vi "HW_Gantner_Parse Construct Default Modu Configuration.vi"(5 "Chan dflt Para in":T5, 7 "DevInfo":T1, 11 "ModuCFG from File":T2) -> (3 "ModuCFG out":T2)   [LabVIEW 2016]
uses:
  Ctrls/HardWare _ Module Configuration.ctl
  Ctrls/HardWare _ Channel Configurations PopUp Type.ctl
  ToolKit/Popup/Private/Ctrls/POP_Data Type.ctl
  Gantner Device Info.ctl
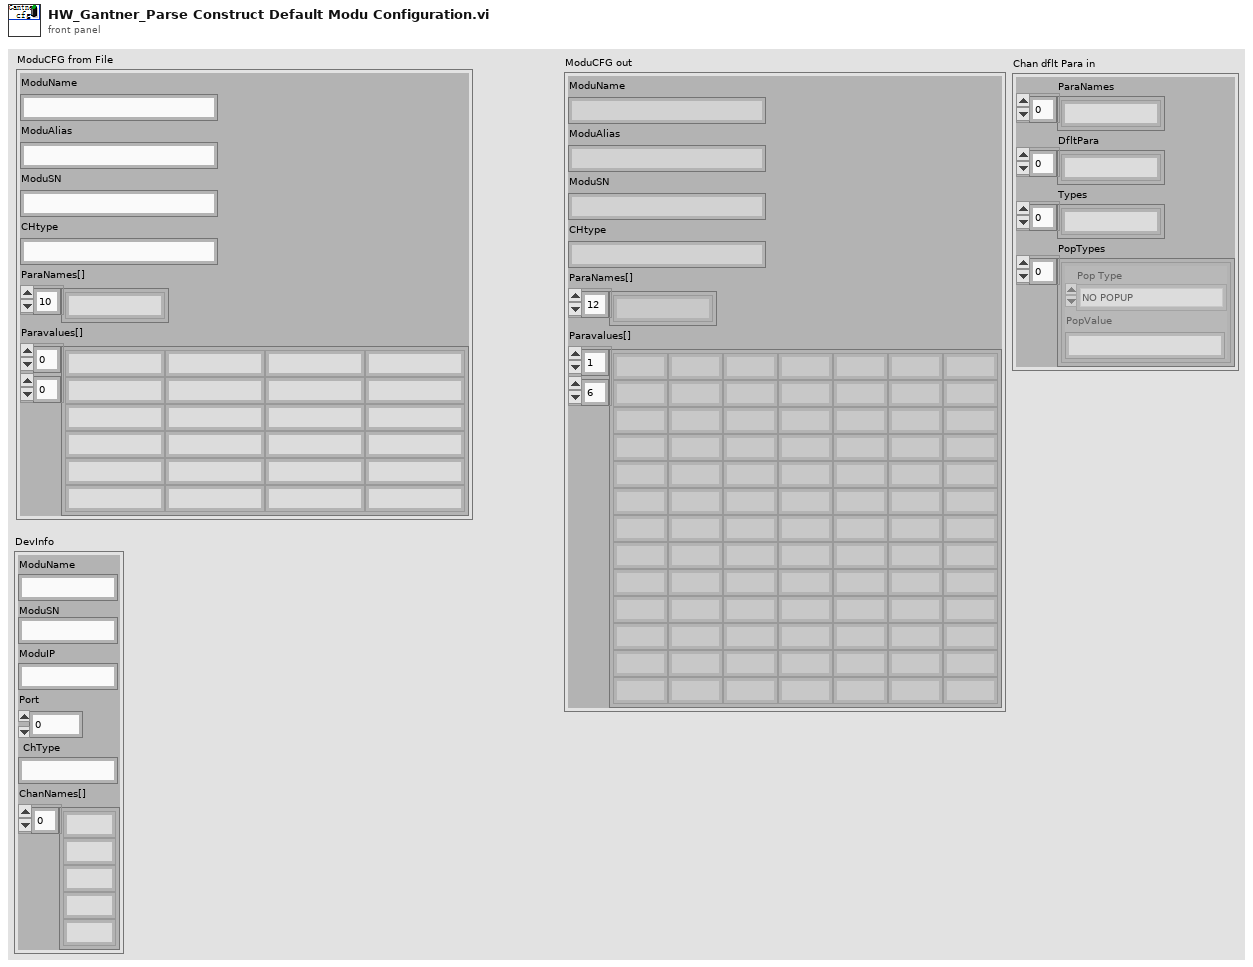
[diagram p1: front panel]
types:
  T1 = typedef "Gantner Device Info.ctl" = cluster{"ModuName":string, "ModuSN":string, "ModuIP":string, "Port":i32, "ChType":string, "ChanNames[]":string[]}
  T2 = typedef "HardWare _ Module Configuration.ctl" = cluster{"ModuName":string, "ModuAlias":string, "ModuSN":string, "CHtype":string, "ParaNames[]":string[], "Paravalues[]":string[][]}
  T3 = typedef "HardWare _ Channel Configurations PopUp Type.ctl" = cluster{"Pop Type":T4, "PopValue":string}
  T4 = typedef "POP_Data Type.ctl" = enum16{"NO POPUP", "Unkown", "String", "Integer", "Float", "Color", "Boolean", "Ring", "Captioned String", "Captioned Integer", "Button Color", "2 Int Cluster", "4 Int Cluster", "6-Dbl Cluster", "Path", "Combox", "Time", "ShotCut String"}
  T5 = cluster{"ParaNames":string[], "DfltPara":string[], "Types":string[], "PopTypes":T3[]}
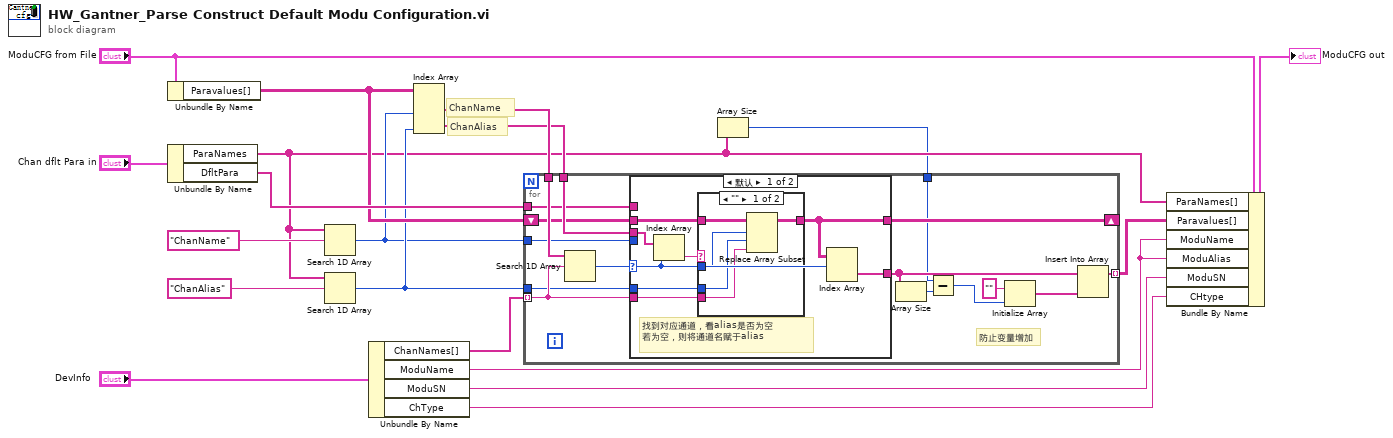
[diagram p0: block diagram]
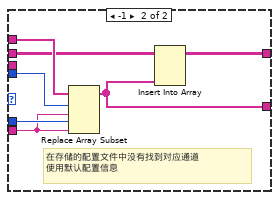
[diagram p3: hidden frame]
diagram:
  # "ChanAlias"
  # "ChanName"
  n1 = Unbundle By Name("ModuCFG from File") -> ("Paravalues[]"=w7:string[][])
  n2 = Unbundle By Name("Chan dflt Para in") -> ("ParaNames"=w2:string[], "DfltPara"=w16:string[])
  n3 = Search 1D Array(1D array=w2, element="ChanName") -> (index of element=w4:i32)  [unwired: 1 in]
  n4 = Search 1D Array(1D array=w2, element="ChanAlias") -> (index of element=w6:i32)  [unwired: 1 in]
  n5 = Unbundle By Name("DevInfo") -> ("ChanNames[]"=w10:string[], "ModuName"=w13:string, "ModuSN"=w12:string, "ChType"=w11:string)
  n6 = Index Array(array=w7, index (col) #1=w4, index (col) #2=w6) -> (element #1=w8:string[], element #2=w5:string[])  [unwired: 2 in]
  n7 = Array Size(array=w2) -> (size(s)=w1:i32)
  n8 = for {
    tunnel: w16 -> [w29]
    tunnel: w6 -> [w27]
    tunnel: w10 -> [w28] mode=indexing
    tunnel: w8 -> [w34]
    tunnel: w5 -> [w33]
    shift-right: [w35] -> _
    shift-left: w7 -> [w31]
    tunnel: w4 -> [w30]
    tunnel: [w26] -> w3 mode=indexing
    tunnel: w1 -> [w23]
    # "防止变量增加"
    n9 = Search 1D Array(1D array=w34, element=w28) -> (index of element=w32:i32)  [unwired: 1 in]
    n10 = case shown="默认" w32 {
      selector: w32 -> [w37 _]
      tunnel: [w38 w51] -> w35
      tunnel: w33 -> [w41 _]
      tunnel: w31 -> [w40 w52]
      tunnel: w30 -> [_ w55]
      tunnel: w29 -> [_ w56]
      tunnel: w28 -> [w42 w53]
      tunnel: w27 -> [w39 w54]
      tunnel: [w36 w50] -> w25
      frame Default {
        # "找到对应通道，看alias是否为空\n若为空，则将通道名赋于alias"
        n11 = Index Array(array=w41, index=w37) -> (element=w43:string)
        n12 = case shown="\"\"" w43 {
          tunnel: w42 -> [w46 _]
          tunnel: w37 -> [w44 _]
          tunnel: w40 -> [w48 w49]
          tunnel: [w45 w49] -> w38
          tunnel: w39 -> [w47 _]
          frame "" {
            n13 = Replace Array Subset(array=w48, new element=w46, index (row)=w44, index (col)=w47) -> (w45:string[][])
          }
          frame Default {
          }
        }
        n14 = Index Array(array=w38, index (row)=w37) -> (element=w36:string[])  [unwired: 1 in]
      }
      frame -1 {
        # "在存储的配置文件中没有找到对应通道\n使用默认配置信息"
        n15 = Replace Array Subset(array=w56, new element #1=w53, index #1=w55, new element #2=w53, index #2=w54) -> (w50:string[])
        n16 = Insert Into Array(array=w52, new element=w50) -> (w51:string[][])  [unwired: 2 in]
      }
    }
    n17 = Array Size(array=w25) -> (size(s)=w24:i32)
    n18 = Subtract(x=w23, y=w24) -> (x-y=w22:i32)
    n19 = Initialize Array("", w22) -> (w20:string[])
    n20 = Insert Into Array(array=w25, new element=w20) -> (w26:string[])  [unwired: 1 in]
  }
  n21 = Bundle By Name(cluster="ModuCFG from File", "ParaNames[]"=w2, "Paravalues[]"=w3, "ModuName"=w13, "ModuAlias"=w13, "ModuSN"=w12, "CHtype"=w11) -> (→"ModuCFG out":T2)
